vi "TFT_Barcode read.vi"(8 "error in":errorcluster, 11 "queue in":refnum<queue>) -> (0 "error out":errorcluster, 1 "exit":bool, 2 "read buffer":string, 3 "queue Out 2":refnum<queue>)   [LabVIEW 2020]
uses:
  Test  enqueue/AutoTest seq.ctl
  <vilib>/Instr/_visa.llb/VISA Configure Serial Port (Instr).vi
  Galobal variable_TI.vi
  Project Setup/Globle Variable/GR_Servo.vi
panel:
  out "x = y?":bool
  out "substring":string
  out "error out 2":errorcluster
  out "error out":errorcluster
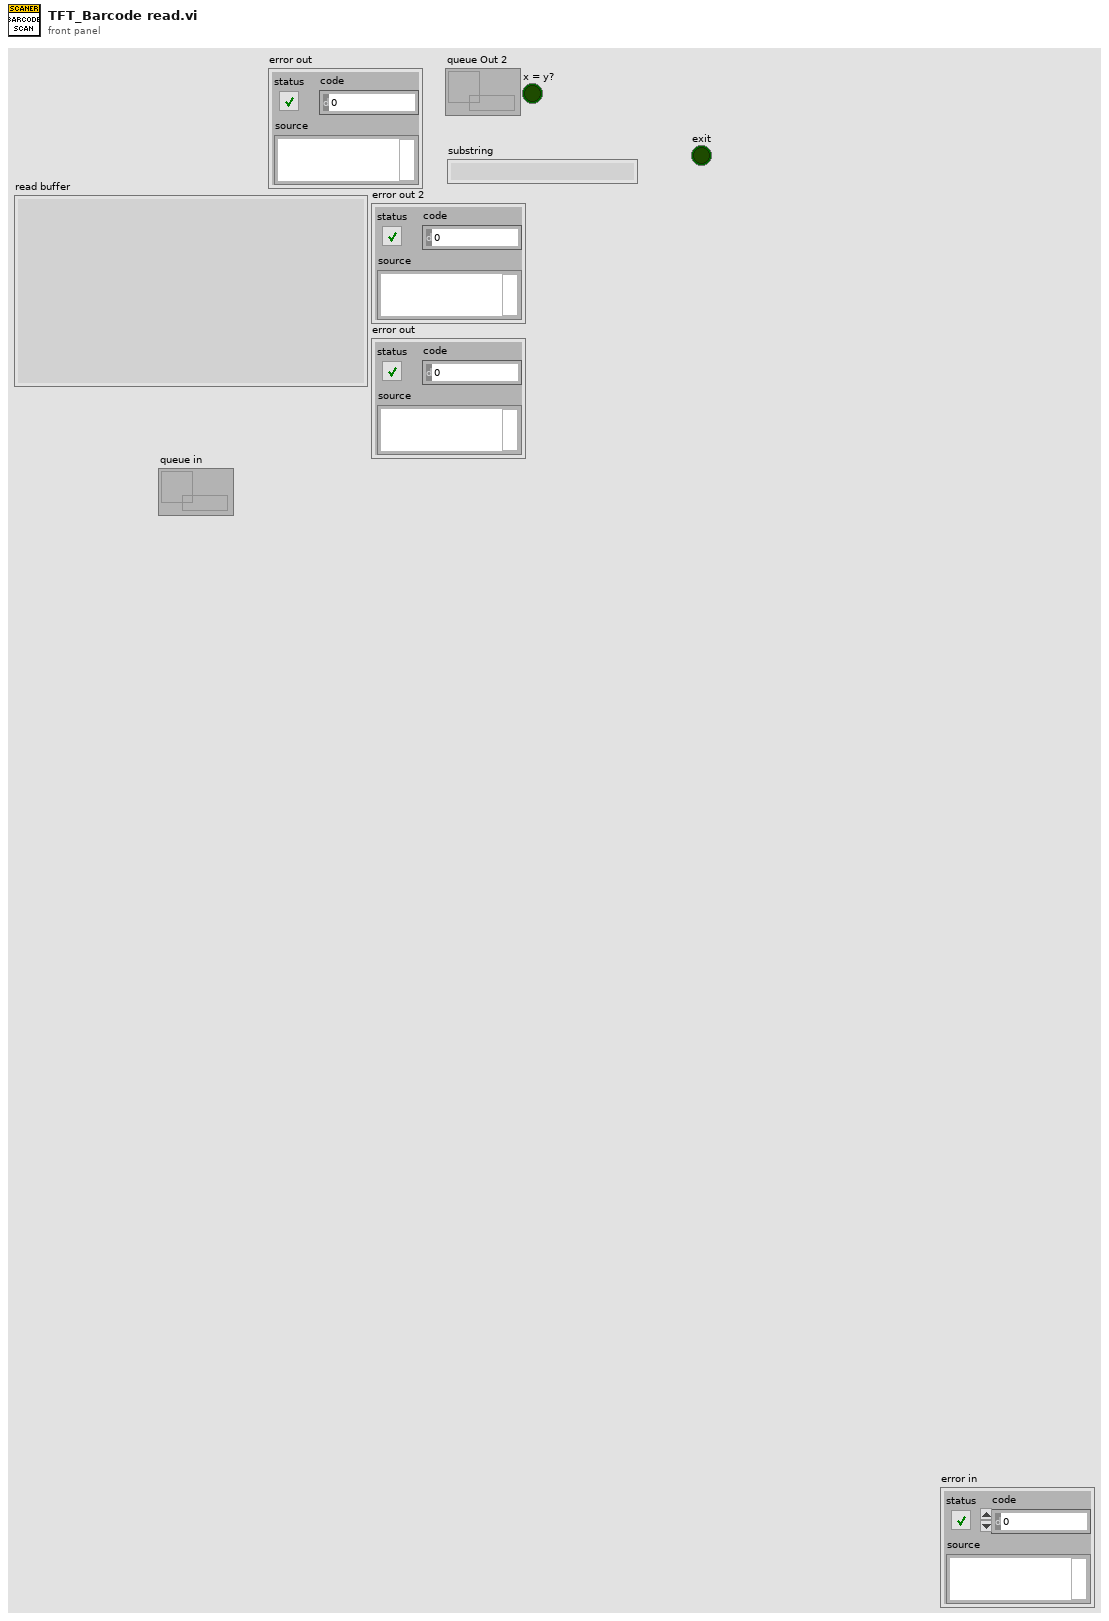
[diagram p1: front panel]
types:
  T1 = cluster{"MaxLoad ":dbl, "Min Load":dbl, "MaxDistance(mm)":dbl, "Min Distance(mm)":dbl, "Load Offset":dbl, "Model":string, "Difusser Code":string, "TFT Code ":string, "LVDT Offset":dbl}
  T2 = cluster{"Start":bool, "Emergency ":bool, "Reset":bool, "Home":bool, "Safety":bool}
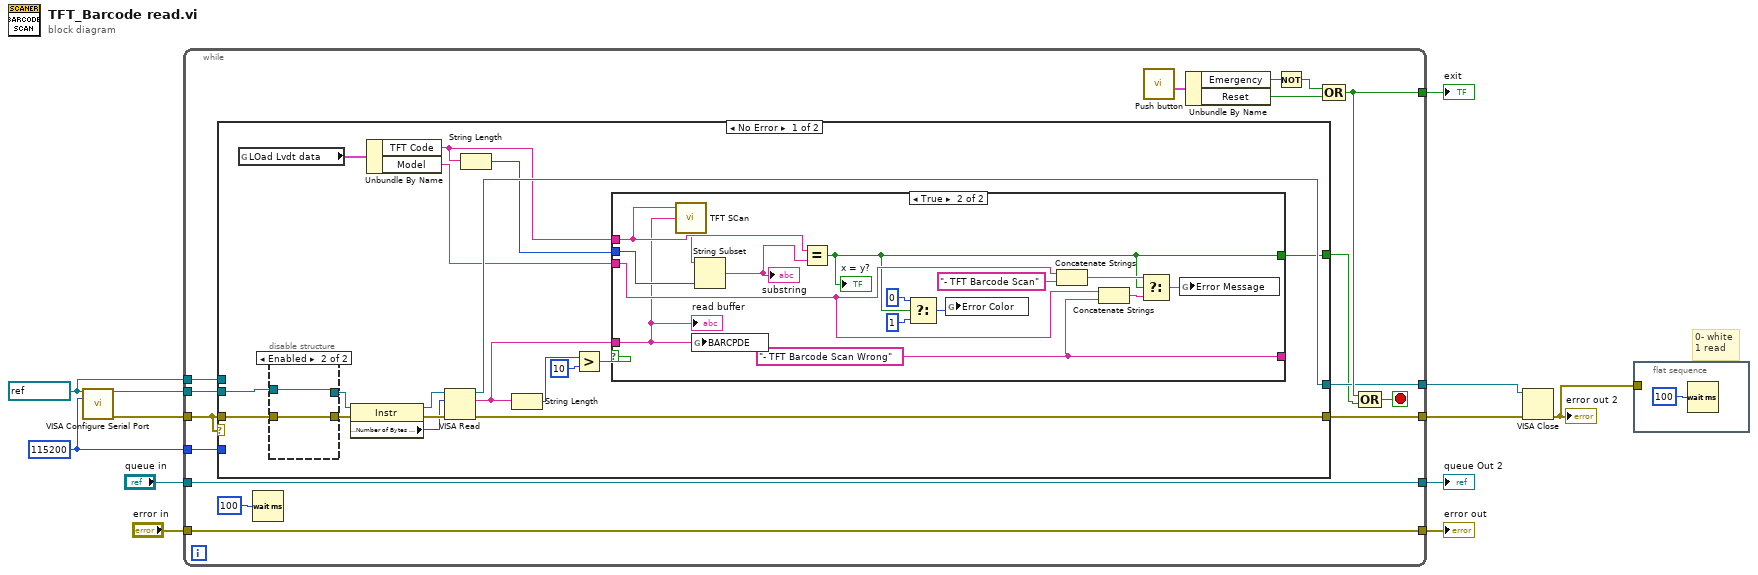
[diagram p0: block diagram]
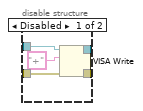
[diagram p2: hidden frame]
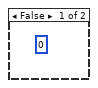
[diagram p3: hidden frame]
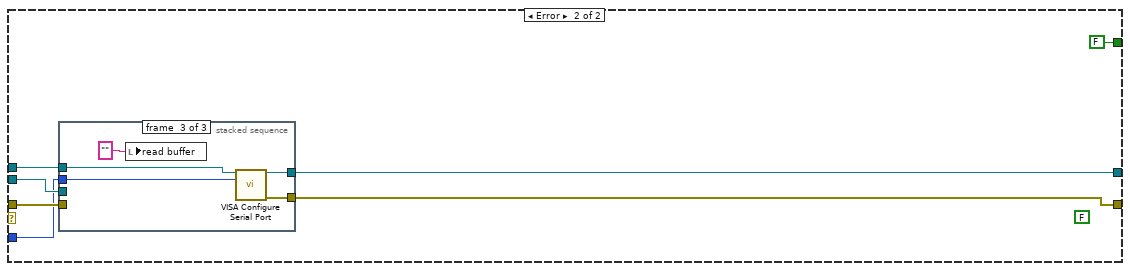
[diagram p4: hidden frame]
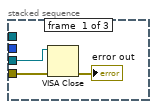
[diagram p5: hidden frame]
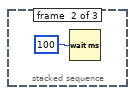
[diagram p6: hidden frame]
diagram:
  w7 = u32 115200 ("baud rate (9600)")
  w8 = refnum<visa-resource-name> "COM1" ("VISA resource name")
  # "0- white\n1 read"
  n1 = call-poly "VISA Configure Serial Port"("VISA resource name"=w8, "baud rate (9600)"=w7) -> ("VISA resource name out"=w12:refnum<visa-resource-name>, "error out"=w11:errorcluster)  [unwired: 12 in]
  n2 = while {
    tunnel: w12 -> [w28]
    tunnel: w11 -> [w26]
    tunnel: [w14] -> w10
    tunnel: [w27] -> w9
    tunnel: w8 -> [w25]
    tunnel: w7 -> [w24]
    tunnel: [w15] -> w6
    tunnel: [w21] -> w4
    tunnel: "queue in" -> [w21]
    tunnel: "error in" -> [w20]
    tunnel: [w20] -> w2
    stop <- w22 stop-if-true
    n3 = case shown="No Error" w26 {
      tunnel: w28 -> [w46 w75]
      tunnel: w26 -> [w45 w74]
      tunnel: [w44 w71] -> w14
      tunnel: [w43 w70] -> w27
      tunnel: w25 -> [_ w73]
      tunnel: w24 -> [_ w72]
      tunnel: [w29 FALSE] -> w13
      frame No Error {
        n4 = global read "Galobal variable_TI.vi" "LOad Lvdt data"() -> (w33:T1)
        n5 = disable-structure shown="Enabled" {
          disable-tunnel: w46 -> [w51 w53]
          disable-tunnel: w45 -> [w50 w52]
          disable-tunnel: [w49 w52] -> w42
          disable-tunnel: [w48 w53] -> w41
          frame Disabled {
            n6 = VISA Write(VISA resource name=w51, write buffer="+", error in (no error)=w50) -> (VISA resource name out=w48:refnum<visa-resource-name>, error out=w49:errorcluster)  [unwired: 1 out]
          }
          frame Enabled {
          }
        }
        n7 = property class="Instr"(reference=w41, error in=w42) -> (reference out=w40:refnum<visa-resource-name>, error out=w39:errorcluster, "Serial Settings:Number of Bytes at Serial Port"=w38:u32)
        n8 = Unbundle By Name(w33) -> ("TFT Code"=w32:string, "Model"=w30:string)
        n9 = VISA Read(VISA resource name=w40, byte count=w38, error in (no error)=w39) -> (VISA resource name out=w44:refnum<visa-resource-name>, read buffer=w35:string, error out=w43:errorcluster)  [unwired: 1 out]
        n10 = String Length(string=w32) -> (length=w31:i32)
        n11 = String Length(string=w35) -> (length=w37:i32)
        n12 = Greater?(x=w37, y=10) -> (0:w34:bool)
        n13 = case shown="True" w34 {
          tunnel: w35 -> [_ w55]
          tunnel: w32 -> [_ w56]
          tunnel: w31 -> [_ w68]
          tunnel: w30 -> [_ w58]
          tunnel: [_ w57] -> w29
          tunnel: [_ w59] -> _
          frame False {
            (unwired) 0 ("f")
          }
          frame True {
            w59 = "- TFT Barcode Scan Wrong" ("string")
            n14 = call "TFT SCan.vi"("Scan Data"=w55, "FTT"=w56) -> ("OutputData"=w54:string)  [unwired: 3 in]
            n15 = global write "Galobal variable_TI.vi" "BARCPDE"(w55) -> ()
            n16 = String Subset(string=w54, length (rest)=w68) -> (substring=w67:string)  [unwired: 1 in]
            "substring" <- w67
            n17 = Equal?(x=w56, y=w67) -> (x = y?=w57:bool)
            "x = y?" <- w57
            n18 = Select(t=0, s=w57, f=1) -> (s? t:f=w64:i32)
            n19 = global write "GR_Servo.vi" "Error Color"(w64) -> ()
            n20 = Concatenate Strings(w58, "- TFT Barcode Scan" ("string")) -> (w62:string)
            n21 = Concatenate Strings(w58, w59) -> (w61:string)
            n22 = Select(t=w62, s=w57, f=w61) -> (s? t:f=w60:string)
            n23 = global write "GR_Servo.vi" "Error Message"(w60) -> ()
            "read buffer" <- w55
          }
        }
      }
      frame Error {
        (unwired) FALSE
        n24 = stacked-sequence {
          tunnel: w75 -> [w77 _ _]
          tunnel: w74 -> [w76 _ _]
          tunnel: w73 -> [_ _ w84]
          tunnel: w72 -> [_ _ w83]
          tunnel: [_ _ w82] -> w71
          tunnel: [_ _ w81] -> w70
          frame #0 {
            n25 = VISA Close(VISA resource name=w77, error in (no error)=w76) -> (error out=→"error out":errorcluster)
          }
          frame #1 {
            n26 = Wait (ms)(milliseconds to wait=u32 100) -> ()  [unwired: 1 out]
          }
          frame #2 {
            n27 = local write "read buffer"("" ("read buffer")) -> ()
            n28 = call-poly "VISA Configure Serial Port"("VISA resource name"=w84, "baud rate (9600)"=w83) -> ("VISA resource name out"=w82:refnum<visa-resource-name>, "error out"=w81:errorcluster)  [unwired: 12 in]
          }
        }
      }
    }
    n29 = Wait (ms)(milliseconds to wait=u32 100) -> ()  [unwired: 1 out]
    n30 = call "Push button.vi"() -> ("Push Button"=w19:T2)  [unwired: 11 in]
    n31 = Unbundle By Name(w19) -> ("Emergency"=w18:bool, "Reset"=w16:bool)
    n32 = Not(x=w18) -> (.not. x?=w17:bool)
    n33 = Compound Arithmetic op=OR(w17, w16) -> (w15:bool)
    n34 = Compound Arithmetic op=OR(w15, w13) -> (w22:bool)
  }
  "exit" <- w6
  "queue Out 2" <- w4
  "error out" <- w2
  n35 = VISA Close(VISA resource name=w10, error in (no error)=w9) -> (error out=w1:errorcluster)
  "error out 2" <- w1
  n36 = flat-sequence {
    tunnel: w1 -> [_]
    frame #0 {
      n37 = Wait (ms)(milliseconds to wait=u32 100) -> ()  [unwired: 1 out]
    }
  }
